vi "Create New Report.vi"(8 "error in (no error)":errorcluster, 9 "Report Path":path, 11 "csv-formatter in":refnum<class "csv-formatter.lvclass">) -> (0 "error out":errorcluster, 3 "csv-formatter out":refnum<class "csv-formatter.lvclass">)   [LabVIEW 2015, in "csv-formatter.lvclass"]
uses:
  csv-formatter.lvclass
  csv-formatter.lvclass/csv-formatter.ctl
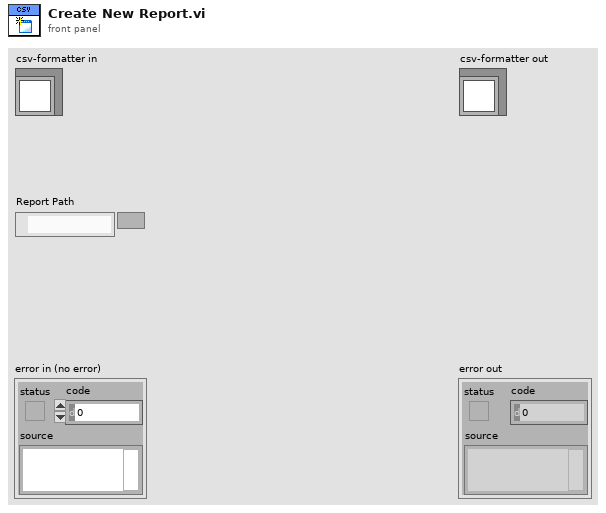
[diagram p1: front panel]
types:
  T1 = typedef "Result Config.ctl" = string[]
  T2 = typedef "Report Header Config.ctl" = string[][]
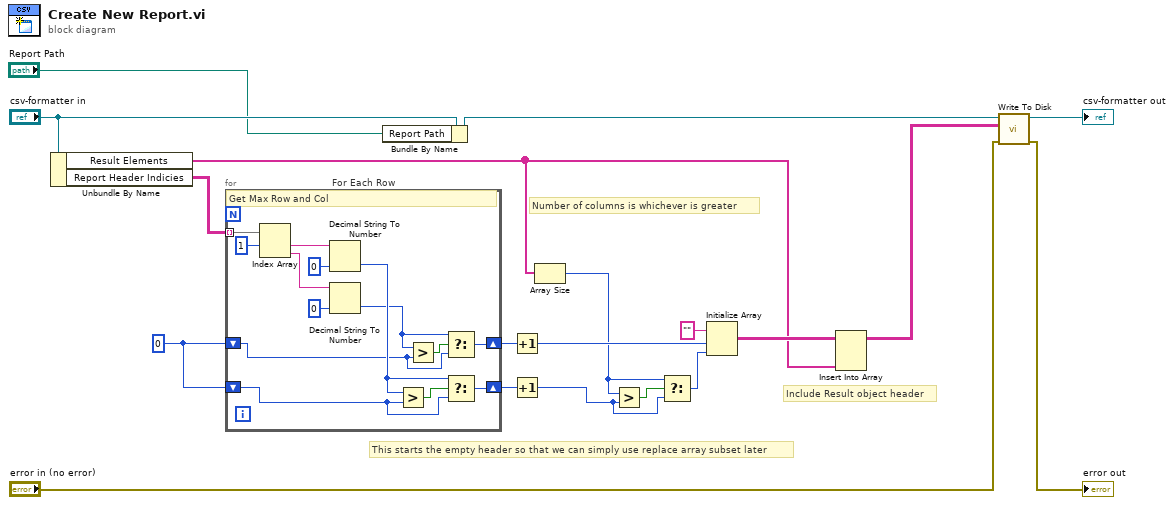
[diagram p0: block diagram]
diagram:
  w18 = 0
  # "Include Result object header"
  # "Number of columns is whichever is greater"
  # "This starts the empty header so that we can simply use replace array subset later"
  n1 = Unbundle By Name("csv-formatter in") -> ("Result Elements"=w7:T1, "Report Header Indicies"=w13:T2)
  n2 = for "For Each Row" {
    shift-right: [w27] -> w16
    shift-left: w18 -> [w21]
    shift-right: [w26] -> w15
    shift-left: w18 -> [w23]
    tunnel: w13 -> [w33] mode=indexing
    # "Get Max Row and Col"
    n3 = Index Array(array=w33, index #1=1 ("index")) -> (element #1=w31:string, element #2=w30:string)  [unwired: 1 in]
    n4 = Decimal String To Number(string=w31, default (0L)=0 ("default (0 I32)")) -> (number=w25:i32)  [unwired: 1 in, 1 out]
    n5 = Decimal String To Number(string=w30, default (0L)=0 ("default (0 I32)")) -> (number=w20:i32)  [unwired: 1 in, 1 out]
    n6 = Greater?(x=w25, y=w23) -> (0:w24:bool)
    n7 = Greater?(x=w20, y=w21) -> (0:w22:bool)
    n8 = Select(t=w20, s=w22, f=w21) -> (s? t:f=w27:i32)
    n9 = Select(t=w25, s=w24, f=w23) -> (s? t:f=w26:i32)
  }
  n10 = Bundle By Name(cluster="csv-formatter in", "Report Path"="Report Path") -> (w2:refnum<class "csv-formatter.lvclass">)
  n11 = Increment(x=w16) -> (x+1=w14:i32)
  n12 = Increment(x=w15) -> (x+1=w10:i32)
  n13 = Array Size(array=w7) -> (size(s)=w11:i32)
  n14 = Greater?(x=w11, y=w10) -> (0:w12:bool)
  n15 = Select(t=w11, s=w12, f=w10) -> (s? t:f=w9:i32)
  n16 = Initialize Array("", w14, w9) -> (w8:string[][])
  n17 = Insert Into Array(array=w8, new element=w7) -> (w5:string[][])  [unwired: 2 in]
  n18 = call "Write To Disk.vi"("error in (no error)"="error in (no error)", "Result In"=w5, "csv-formatter in"=w2) -> ("error out"=→"error out":errorcluster, "csv-formatter out"=→"csv-formatter out":refnum<class "csv-formatter.lvclass">)  [unwired: 7 in]
